vi "writeNotification.vi"(7 "string":string, 8 "Array":T1) -> ()   [LabVIEW 2017]
uses:
  RefArray/RefArray.ctl
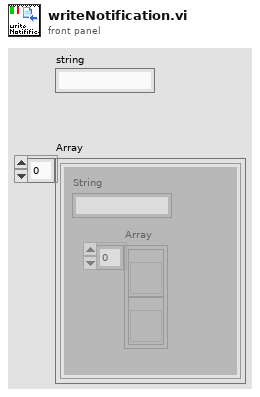
[diagram p1: front panel]
types:
  T1 = typedef "RefArray.ctl" = cluster{"String":string, "Array":refnum<vi>[]}[]
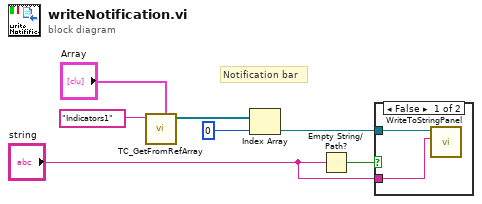
[diagram p0: block diagram]
diagram:
  # "Notification bar"
  n1 = call "TC_GetFromRefArray.vi"("arrayIn"="Array", "NameToFind"="Indicators1") -> ("refArray"=w4:refnum<vi>[])  [unwired: 8 in, 1 out]
  n2 = Index Array(array=w4, index=0) -> (element=w3:refnum<vi>)
  n3 = Empty String/Path?(string/path="string") -> (empty?=w2:bool)
  n4 = case shown="False" w2 {
    tunnel: w3 -> [w9 _]
    tunnel: "string" -> [w8 _]
    frame False {
      n5 = call "WriteToStringPanel.vi"("String"=w8, "Ctl Refnum"=w9) -> ()  [unwired: 10 in]
    }
    frame True {
    }
  }
